vi "IpConfig.vi"(0 "Gateway":string caption="修改网关", 1 "SubnetMask":string caption="修改子网掩码", 2 "IP":string caption="修改IP地址", 3 "CurrentIP":string caption="原始IP地址") -> ()   [LabVIEW 2012]
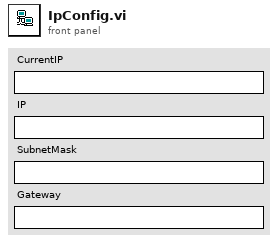
[diagram p1: front panel]
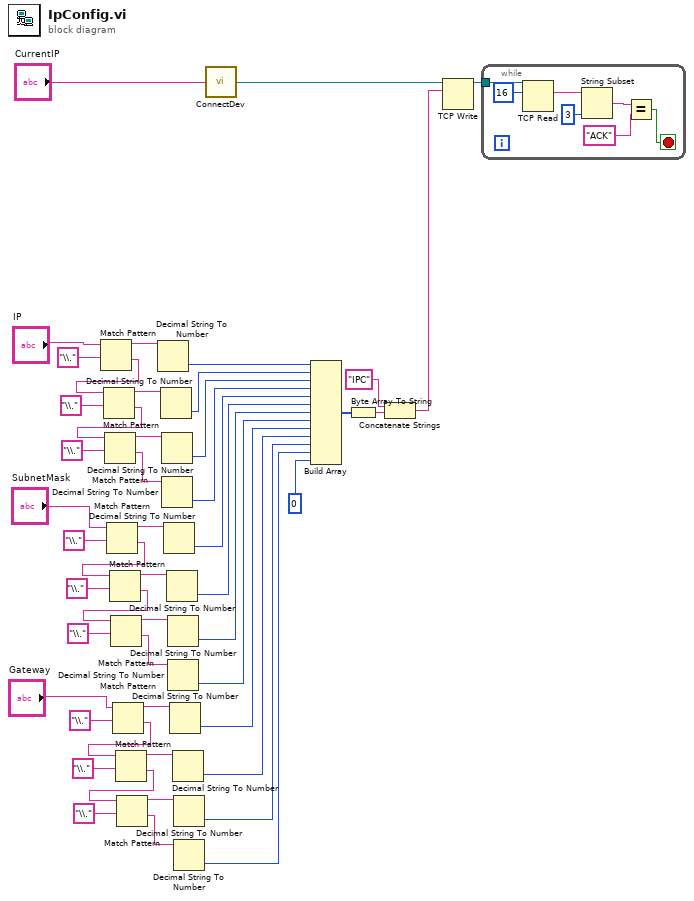
[diagram p0: block diagram]
diagram:
  n1 = Match Pattern(string="IP", regular expression="\\.") -> (before substring=w45:string, after substring=w40:string)  [unwired: 1 in, 2 out]
  n2 = Match Pattern(string=w40, regular expression="\\.") -> (before substring=w43:string, after substring=w39:string)  [unwired: 1 in, 2 out]
  n3 = Match Pattern(string=w39, regular expression="\\.") -> (before substring=w41:string, after substring=w38:string)  [unwired: 1 in, 2 out]
  n4 = Match Pattern(string="SubnetMask", regular expression="\\.") -> (before substring=w36:string, after substring=w31:string)  [unwired: 1 in, 2 out]
  n5 = Match Pattern(string=w31, regular expression="\\.") -> (before substring=w34:string, after substring=w30:string)  [unwired: 1 in, 2 out]
  n6 = Match Pattern(string=w30, regular expression="\\.") -> (before substring=w32:string, after substring=w29:string)  [unwired: 1 in, 2 out]
  n7 = Match Pattern(string="Gateway", regular expression="\\.") -> (before substring=w27:string, after substring=w22:string)  [unwired: 1 in, 2 out]
  n8 = Match Pattern(string=w22, regular expression="\\.") -> (before substring=w25:string, after substring=w21:string)  [unwired: 1 in, 2 out]
  n9 = Match Pattern(string=w21, regular expression="\\.") -> (before substring=w23:string, after substring=w20:string)  [unwired: 1 in, 2 out]
  n10 = Decimal String To Number(string=w45) -> (number=w3:i32)  [unwired: 2 in, 1 out]
  n11 = Decimal String To Number(string=w43) -> (number=w4:i32)  [unwired: 2 in, 1 out]
  n12 = Decimal String To Number(string=w41) -> (number=w5:i32)  [unwired: 2 in, 1 out]
  n13 = Decimal String To Number(string=w38) -> (number=w6:i32)  [unwired: 2 in, 1 out]
  n14 = Decimal String To Number(string=w36) -> (number=w7:i32)  [unwired: 2 in, 1 out]
  n15 = Decimal String To Number(string=w34) -> (number=w8:i32)  [unwired: 2 in, 1 out]
  n16 = Decimal String To Number(string=w32) -> (number=w9:i32)  [unwired: 2 in, 1 out]
  n17 = Decimal String To Number(string=w29) -> (number=w10:i32)  [unwired: 2 in, 1 out]
  n18 = Decimal String To Number(string=w27) -> (number=w11:i32)  [unwired: 2 in, 1 out]
  n19 = Decimal String To Number(string=w25) -> (number=w12:i32)  [unwired: 2 in, 1 out]
  n20 = Decimal String To Number(string=w23) -> (number=w13:i32)  [unwired: 2 in, 1 out]
  n21 = Decimal String To Number(string=w20) -> (number=w14:i32)  [unwired: 2 in, 1 out]
  n22 = call "ConnectDev.vi"("IP."="CurrentIP") -> ("connection ID"=w2:refnum<k5>)
  n23 = Build Array(w3, w4, w5, w6, w7, w8, w9, w10, w11, w12, w13, w14, 0 ("元素")) -> (w16:i32[])
  n24 = Byte Array To String(unsigned byte array=w16) -> (string=w19:string)
  n25 = Concatenate Strings("IPC" ("数据输入"), w19) -> (w17:string)
  n26 = TCP Write(connection ID=w2, data in=w17) -> (connection ID out=w47:refnum<k5>)  [unwired: 2 in, 2 out]
  n27 = while {
    tunnel: w47 -> [w57]
    stop <- w52 stop-if-true
    n28 = TCP Read(connection ID=w57, bytes to read=16 ("读取的字节")) -> (data out=w55:string)  [unwired: 3 in, 2 out]
    n29 = String Subset(string=w55, length (rest)=3 ("偏移量(0)")) -> (substring=w54:string)  [unwired: 1 in]
    n30 = Equal?(x=w54, y="ACK") -> (x = y?=w52:bool)
  }
